vi "PID Loop SubVI.vi"(6 "reinitialize? (F)":bool, 8 "Output Limits":cluster{"Max":dbl, "Min":dbl}, 9 "Measured Flowrate":dbl[](array[numeric]), 10 "Desired Flowrate":dbl[](array[numeric]), 11 "Gains":T1(array[cluster])) -> (3 "Array out":dbl[](array[numeric]))   [LabVIEW 2021]
uses:
  <vilib>/addons/control/pid/pid.llb/PID (DBL).vi
  <vilib>/addons/control/pid/NI_PID_pid.lvlib
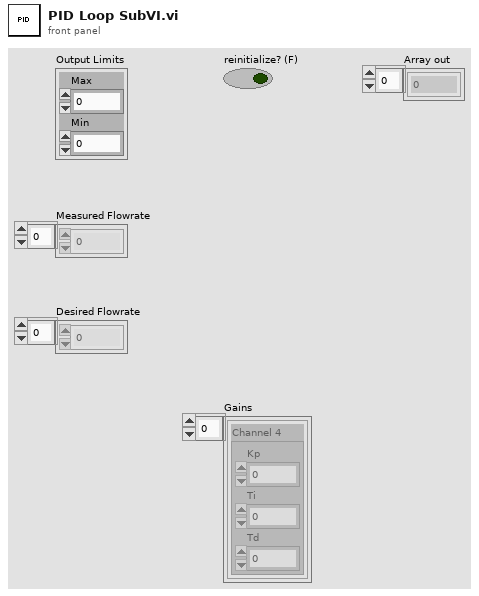
[diagram p1: front panel]
types:
  T1 = cluster{"Channel 4":cluster{"Kp":dbl, "Ti":dbl, "Td":dbl}}[]
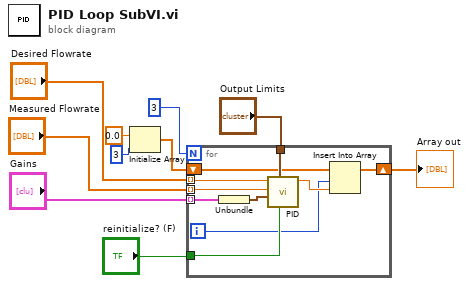
[diagram p0: block diagram]
diagram:
  n1 = Initialize Array(0.0 ("element"), 3 ("dimension size")) -> (w6:dbl[])
  n2 = for {
    N: 3 -> [_]
    tunnel: "Measured Flowrate" -> [w11] mode=indexing
    tunnel: "Desired Flowrate" -> [w20] mode=indexing
    tunnel: "Gains" -> [w19] mode=indexing
    tunnel: "Output Limits" -> [w17]
    tunnel: "reinitialize? (F)" -> [w16]
    shift-right: [w14] -> w10
    shift-left: w6 -> [w13]
    i -> [w12]
    n3 = Unbundle(w19) -> ("Channel 4"=w18:cluster{"Kp":dbl, "Ti":dbl, "Td":dbl})
    n4 = call-poly <vilib>:"PID.vi"("reinitialize? (F)"=w16, "output range"=w17, "PID gains"=w18, "process variable"=w11, "setpoint"=w20) -> ("output"=w15:dbl)  [unwired: 5 in, 1 out]
    n5 = Insert Into Array(array=w13, index=w12, new element=w15) -> (w14:dbl[])
  }
  "Array out" <- w10
